vi "GetDriveRefnum.vi"() -> (2 "RobotDriveDevRef":T1={"DevStatus"={"status"=FALSE, "code"=0, "source"=""}, "Motors[]"=[], "Square Inputs"=FALSE, "Max Output"=1.0}, 3 "RobotDriveDevRef 2":T1={"DevStatus"={"status"=FALSE, "code"=0, "source"=""}, "Motors[]"=[], "Square Inputs"=FALSE, "Max Output"=1.0})   [LabVIEW 2016, in "DriveBase.lvclass"]
uses:
  DriveBase.lvclass
  <vilib>/Rock Robotics/WPI/RobotDrive/WPI_RobotDriveDevRef.ctl
  <vilib>/Rock Robotics/WPI/MotorControl/WPI_MotorControlDeviceRef.ctl
  <vilib>/Rock Robotics/WPI/MotorControl/WPI_MotorControlType.ctl
  <vilib>/Rock Robotics/SystemInterfaces/DIO/FPGA_DIOPWMChannel.ctl
  <vilib>/Rock Robotics/WPI/PWM/WPI_PWMDeadband.ctl
  <vilib>/Rock Robotics/WPI/Utilities/WPI_GetSetVariantRefNum.vi
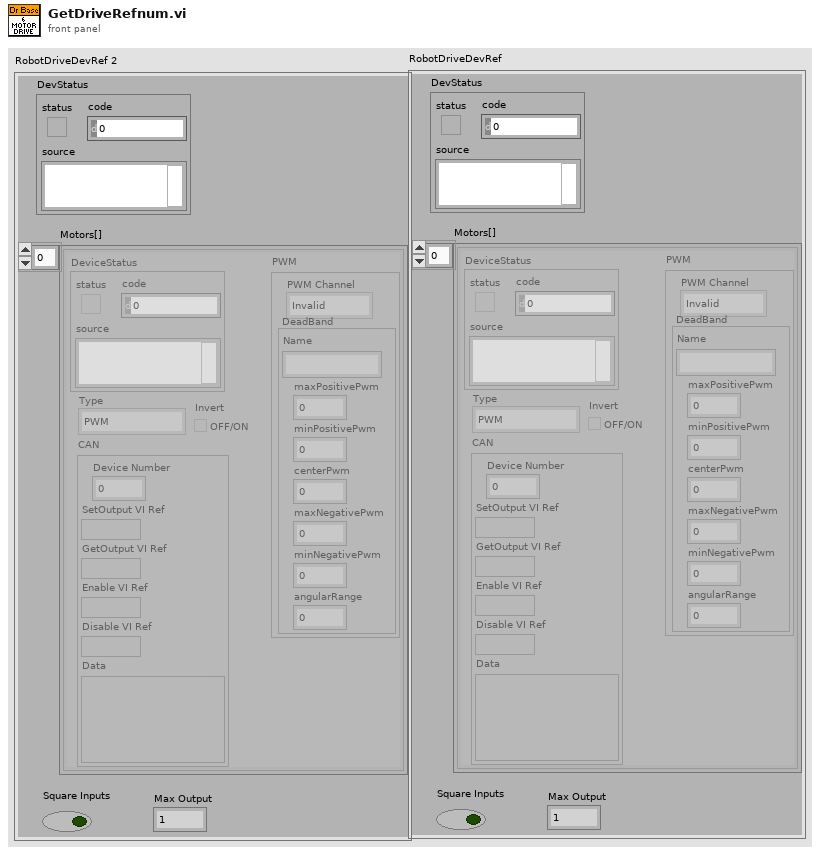
[diagram p1: front panel]
types:
  T1 = typedef "WPI_RobotDriveDevRef.ctl" = cluster{"DevStatus":errorcluster, "Motors[]":T2[], "Square Inputs":bool, "Max Output":dbl}
  T2 = typedef "WPI_MotorControlDeviceRef.ctl" = cluster{"DeviceStatus":errorcluster, "Type":T3, "PWM":cluster{"PWM Channel":T4, "DeadBand":T5}, "CAN":cluster{"Device Number":u8, "SetOutput VI Ref":variant, "GetOutput VI Ref":variant, "Enable VI Ref":variant, "Disable VI Ref":variant, "Data":variant}, "Invert":bool}
  T3 = typedef "WPI_MotorControlType.ctl" = enum16{"PWM", "CAN"}
  T4 = typedef "FPGA_DIOPWMChannel.ctl" = enum8{"PWM 0", "PWM 1", "PWM 2", "PWM 3", "PWM 4", "PWM 5", "PWM 6", "PWM 7", "PWM 8", "PWM 9", "PWM MXP 0", "PWM MXP 1", "PWM MXP 2", "PWM MXP 3", "PWM MXP 4", "PWM MXP 5", "PWM MXP 6", "PWM MXP 7", "PWM MXP 8", "PWM MXP 9", "Invalid"}
  T5 = typedef "WPI_PWMDeadband.ctl" = cluster{"Name":string, "maxPositivePwm":i32, "minPositivePwm":i32, "centerPwm":i32, "maxNegativePwm":i32, "minNegativePwm":i32, "angularRange":u16}
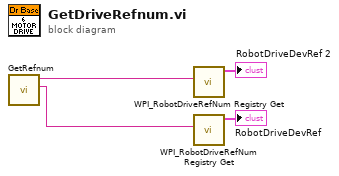
[diagram p0: block diagram]
diagram:
  n1 = call "GetRefnum.vi"() -> ("RobotDriveRefnum1"=w3:string, "RobotDriveRefnum2"=w4:string)  [unwired: 9 in, 1 out]
  n2 = call <vilib>:"WPI_RobotDriveRefNum Registry Get.vi"("refnum name"=w4) -> ("RobotDriveDevRef"=→"RobotDriveDevRef 2":T1)  [unwired: 9 in, 1 out]
  n3 = call <vilib>:"WPI_RobotDriveRefNum Registry Get.vi"("refnum name"=w3) -> ("RobotDriveDevRef"=→"RobotDriveDevRef":T1)  [unwired: 9 in, 1 out]
